vi "Dilution_visible.vi"(1 "calculated":u16, 2 "dilution":bool) -> (0 "Visible":T1)   [LabVIEW 2011]
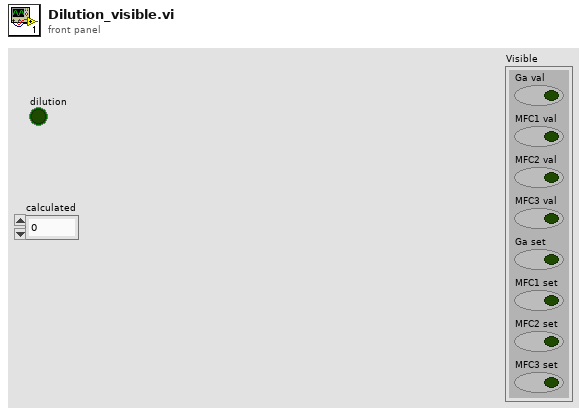
[diagram p1: front panel]
types:
  T1 = cluster{"Ga val":bool, "MFC1 val":bool, "MFC2 val":bool, "MFC3 val":bool, "Ga set":bool, "MFC1 set":bool, "MFC2 set":bool, "MFC3 set":bool}
  T2 = cluster{"Visible":bool, "Visible":bool, "Visible":bool, "Visible":bool, "Visible":bool, "Visible":bool, "Visible":bool, "Visible":bool}
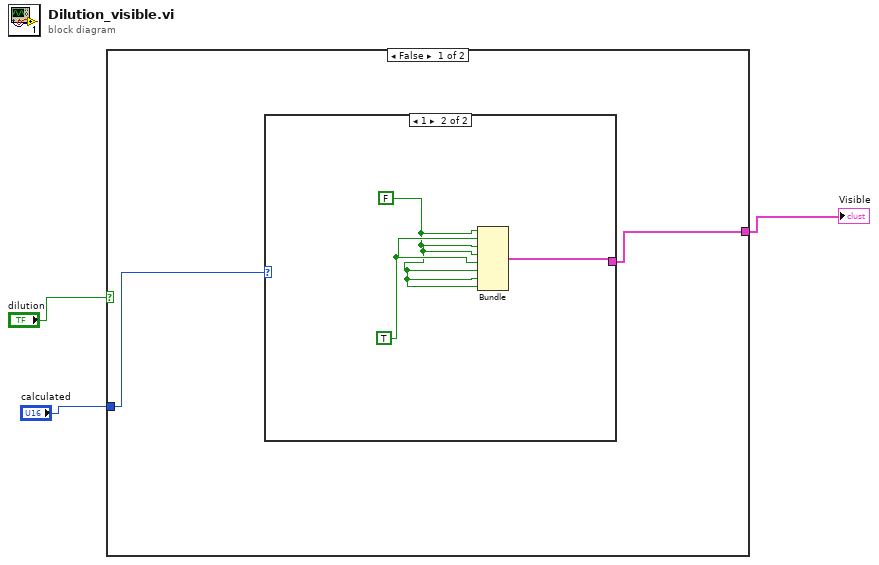
[diagram p0: block diagram]
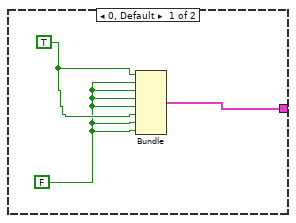
[diagram p2: hidden frame]
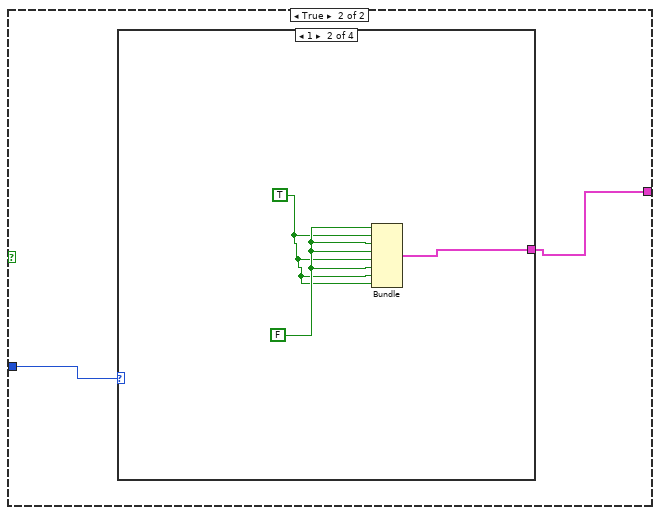
[diagram p3: hidden frame]
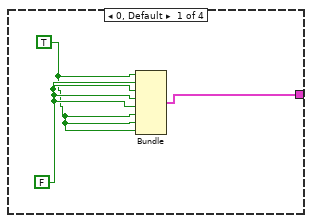
[diagram p4: hidden frame]
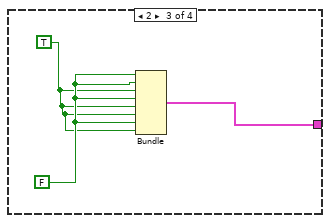
[diagram p5: hidden frame]
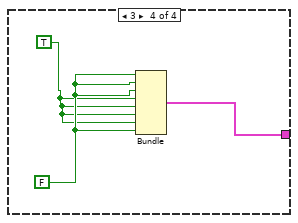
[diagram p6: hidden frame]
diagram:
  n1 = case shown="False" "dilution" {
    tunnel: [w5 w13] -> w2
    tunnel: "calculated" -> [w4 w12]
    frame False {
      n2 = case shown="1" w4 {
        tunnel: [w7 w11] -> w5
        frame 0, Default {
          w6 = FALSE ("Visible")
          w8 = TRUE ("Visible")
          n3 = Bundle("Visible"=w8, "Visible"=w6, "Visible"=w6, "Visible"=w6, "Visible"=w6, "Visible"=w8, "Visible"=w6, "Visible"=w6) -> (w7:T2)  [unwired: 1 in]
        }
        frame 1 {
          w10 = TRUE ("Visible")
          w9 = FALSE ("Visible")
          n4 = Bundle("Visible"=w9, "Visible"=w10, "Visible"=w9, "Visible"=w9, "Visible"=w10, "Visible"=w9, "Visible"=w9, "Visible"=w9) -> (w11:T2)  [unwired: 1 in]
        }
      }
    }
    frame True {
      n5 = case shown="1" w12 {
        tunnel: [w14 w17 w22 w25] -> w13
        frame 0, Default {
          w16 = FALSE ("Visible")
          w15 = TRUE ("Visible")
          n6 = Bundle("Visible"=w15, "Visible"=w16, "Visible"=w16, "Visible"=w16, "Visible"=w16, "Visible"=w15, "Visible"=w15, "Visible"=w15) -> (w14:T2)  [unwired: 1 in]
        }
        frame 1 {
          w19 = FALSE ("Visible")
          w18 = TRUE ("Visible")
          n7 = Bundle("Visible"=w19, "Visible"=w18, "Visible"=w19, "Visible"=w19, "Visible"=w18, "Visible"=w19, "Visible"=w18, "Visible"=w18) -> (w17:T2)  [unwired: 1 in]
        }
        frame 2 {
          w21 = FALSE ("Visible")
          w20 = TRUE ("Visible")
          n8 = Bundle("Visible"=w21, "Visible"=w21, "Visible"=w20, "Visible"=w21, "Visible"=w20, "Visible"=w20, "Visible"=w21, "Visible"=w20) -> (w22:T2)  [unwired: 1 in]
        }
        frame 3 {
          w24 = FALSE ("Visible")
          w23 = TRUE ("Visible")
          n9 = Bundle("Visible"=w24, "Visible"=w24, "Visible"=w24, "Visible"=w23, "Visible"=w23, "Visible"=w23, "Visible"=w23, "Visible"=w24) -> (w25:T2)  [unwired: 1 in]
        }
      }
    }
  }
  "Visible" <- w2
